vi "Factory Create.vi"(8 "Error In":errorcluster, 11 "reference in":refnum<class "Voltmeter Virtual CFG.lvclass">) -> (0 "Error Out":errorcluster, 3 "reference out":refnum<class "Voltmeter Virtual CFG.lvclass">)   [LabVIEW 2023, in "Voltmeter Virtual.lvlib" / "Voltmeter Virtual CFG.lvclass"]
uses:
  Voltmeter Virtual CFG.lvclass
  Voltmeter Virtual CFG.lvclass/Voltmeter Virtual CFG.ctl
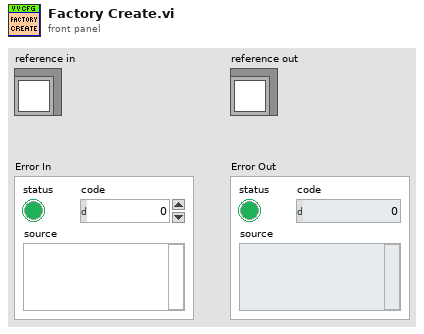
[diagram p1: front panel]
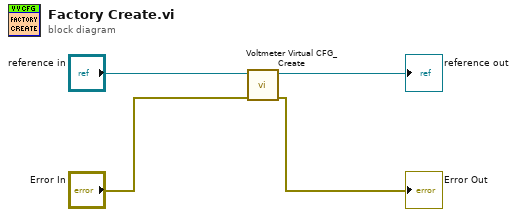
[diagram p0: block diagram]
diagram:
  n1 = call "Voltmeter Virtual CFG_Create.vi"("Error In"="Error In", "reference in"="reference in") -> ("Error Out"=→"Error Out":errorcluster, "reference out"=→"reference out":refnum<class "Voltmeter Virtual CFG.lvclass">)  [unwired: 8 in]
